vi "LIN framegen.vi"(11 "OOB to Logic Data in":T3 {"Payload LIN" format="%x"; "ID LIN" format="%x"; "Payload CAN" format="%x"; "Type CAN" items=["CAN Data"=0, "CAN Remote"=1, "CAN Bus Error"=2, "CAN 2.0 Data"=8, "CAN FD Data"=16, "CAN FD+BRS Data"=24, "J1939 Data"=192, "Delay"=224, "Log Trigger"=225, "Start Trigger"=226]; "ID CAN" format="%x"}) -> (2 "DLC 2":u32, 3 "Array":T1[](array[typedef]) {"event ID" format="%x"; "payload" format="%x"; "timestamp" format="%<%.7X\n%x>T"; "type" items=["LIN Data"=64, "LIN Bus Error"=65, "LIN No Response"=66, "Delay"=224, "Log Trigger"=225, "Start Trigger"=226]; "identifier" format="%x"})   [LabVIEW 2025, in "CAN-LIN Frame Generator.lvclass"]
uses:
  CAN-LIN Frame Generator.lvclass
  CAN-LIN Frame Generator.lvclass/CAN-LIN Frame Generator.ctl
  <vilib>/xnet/xnet.llb/XNET Frame Type LIN.ctl
  <vilib>/xnet/xnet.llb/XNET Frame LIN.ctl
  <vilib>/xnet/xnet.llb/XNET Frame Type CAN.ctl
  OOB Data Transfer/Typdefs/OOB to Logic Data.ctl
  OOB Data Transfer/OOB Data Transfer.lvlib
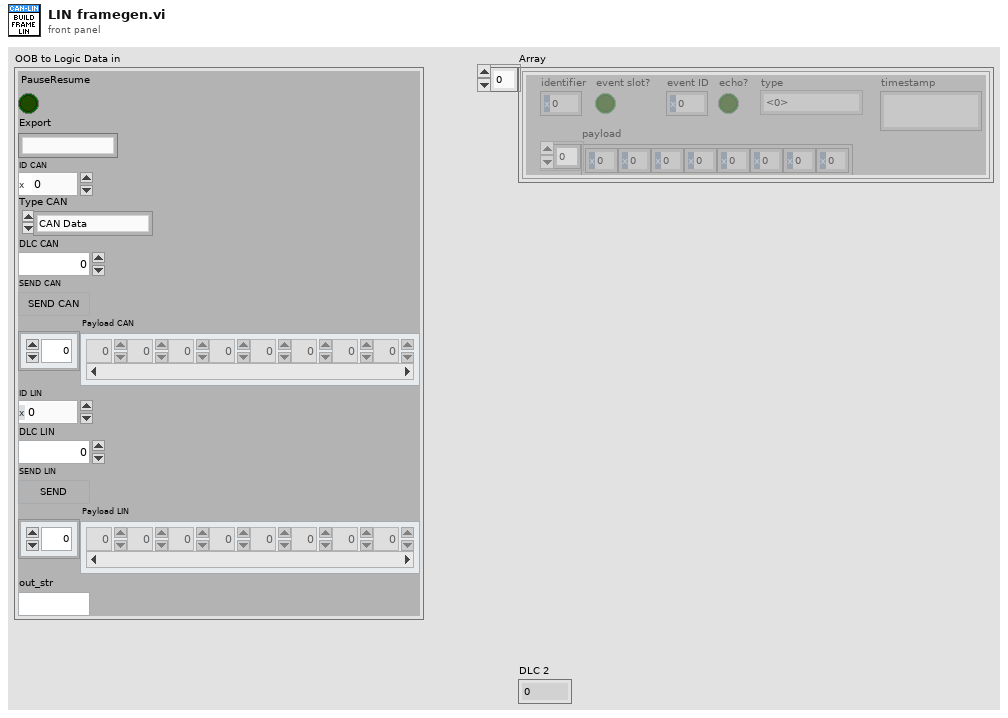
[diagram p1: front panel]
types:
  T1 = typedef "XNET Frame LIN.ctl" = cluster{"timestamp":timestamp, "payload":u8[], "identifier":u32, "type":T2, "event ID":u8, "event slot?":bool, "echo?":bool}
  T2 = typedef "XNET Frame Type LIN.ctl" = u8
  T3 = typedef "OOB Data Transfer.lvlib/OOB to Logic Data.ctl" = cluster{"PauseResume":bool, "Export":string, "ID CAN":u32, "Type CAN":T4, "DLC CAN":u32, "SEND CAN":bool, "Payload CAN":u32[], "ID LIN":u32, "DLC LIN":u32, "SEND LIN":bool, "Payload LIN":u32[], "out_str":string}
  T4 = typedef "XNET Frame Type CAN.ctl" = u8
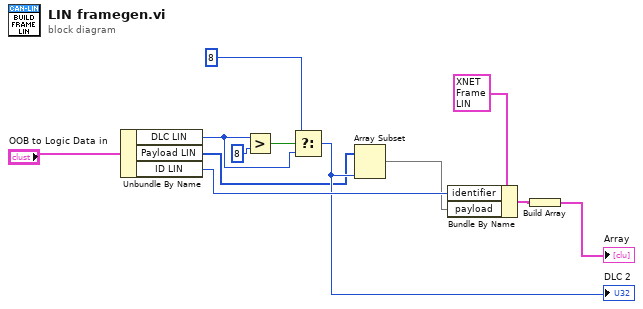
[diagram p0: block diagram]
diagram:
  n1 = Unbundle By Name("OOB to Logic Data in") -> ("DLC LIN"=w9:u32, "Payload LIN"=w10:u32[], "ID LIN"=w12:u32)
  n2 = Greater?(x=w9, y=u32 8) -> (0:w5:bool)
  n3 = Select(t=u32 8, s=w5, f=w9) -> (s? t:f=w11:u32)
  "DLC 2" <- w11
  n4 = Array Subset(array=w10, length=w11) -> (w7:u32[])  [unwired: 1 in]
  n5 = Bundle By Name(cluster=T1 {"timestamp"=timestamp(0 s since 1904-01-01), "payload"=[0, 0, 0, 0, 0, 0, 0, 0], "identifier"=0, "type"=64, "event ID"=0, "event slot?"=FALSE, "echo?"=FALSE} ("LIN frame"), "identifier"=w12, "payload"=w7) -> (w2:T1)
  n6 = Build Array(w2) -> (→"Array":T1[])
